vi "PH_PILS.set PPMA.vi"(0 "i ref in":refnum<vi>, 2 "Tagname":string="N/A", 5 "error in":errorcluster) -> (14 "i ref out":refnum<vi>, 19 "error out":errorcluster)   [LabVIEW 2014, in "PH_PILS.lvlib"]
doc: "Sets GUI elements related to PPMA."
uses:
  PH_PILS.lvlib
  PH_Common/PH_Common.lvlib
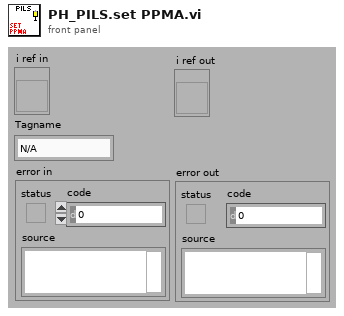
[diagram p1: front panel]
types:
  T1 = typedef "PH_PILS.lvlib/PH_PILS.i attribute.ctl" = cluster{"Boolean":cluster{"GUI Ref":refnum<vi>, "Status":i32}[], "GUI Refs Exp. Shutters":cluster{"1":refnum<vi>, "2":refnum<vi>, "3":refnum<vi>, "4":refnum<vi>}, "Tristate2Run GUI Refs":refnum<vi>[], "EO-Likes":cluster{"GUI Ref":refnum<vi>, "Status":i32}[], "Operation Mode":cluster{"Operation Mode":T2, "GUI":cluster{"Ref State":refnum<vi>, "Ref":refnum<vi>}, "Servicemode":cluster{"Tagname":string, "Status":i32}, "Labormode":cluster{"Tagname":string, "Status":i32}, "Searchmode":cluster{"Tagname":string, "Status":i32}, "Shotmode":cluster{"Tagname":string, "Status":i32}}, "Submode":cluster{"Submode":T3, "GUI":cluster{"Ref State":refnum<vi>, "Ref":refnum<vi>}, "Submode":cluster{"Tagname":string, "Status":i32}}, "Experiment":cluster{"Experiment":enum16{"unknown", "intern", "4 (Z6)", "3", "2", "1"}, "GUI":cluster{"Ref State":refnum<vi>, "Ref":refnum<vi>}, "intern":cluster{"Tagname":string, "Status":i32}, "Exp 4":cluster{"Tagname":string, "Status":i32}, "Exp 3":cluster{"Tagname":string, "Status":i32}, "Exp 2":cluster{"Tagname":string, "Status":i32}, "Exp 1":cluster{"Tagname":string, "Status":i32}}, "TristateNormal":cluster{"GUI Ref":refnum<vi>, "Status":i32}[], "Door Tags":cluster{"GUI Ref":refnum<vi>, "Status":i32}[], "GUIlessTags":cluster{"Name":string, "Status":i32}[], "Beamline GUI Refs":refnum<vi>[], "Special Boolean":cluster{"GUI Ref":refnum<vi>, "Status":i32}[], "Laserpower":cluster{"GUI Ref":refnum<vi>, "Status":i32}[], "Shutter":cluster{"GUI Ref":refnum<vi>, "Status":i32}[], "Tristate EO Like":cluster{"GUI Ref":refnum<vi>, "Status":i32}[], "PP":cluster{"GUI Ref":refnum<vi>, "Status":i32, "Head Ref":refnum<vi>, "Slider Ref":refnum<vi>}[], "Switch Knobs":cluster{"GUI Ref":refnum<vi>, "Status":i32}[], "Latch Knob GUI Refs":refnum<vi>[], "FailureCounter":i32, "Enabled Status":cluster{"Laser":i32, "PreAmp":i32, "MainAmp":i32}, "Mercury":refnum<vi>, "Instance Rods":string, "Logfile":path, "Beckhoff-Instance Internal":string, "Beckhoff-Instance External":string, "Enabling Rights":cluster{"Name":string, "Password":string, "PA?":bool, "MA?":bool, "Exp?":bool}[]}
  T2 = typedef "PH_PILS.lvlib/PH_PILS.Operation Mode.ctl" = enum16{"unknown", "Service", "Labor", "Search", "Shot"}
  T3 = typedef "PH_PILS.lvlib/PH_PILS.Submode.ctl" = enum16{"unknown", "HV-Normal", "HV-Test"}
  T4 = cluster{"GUI Ref":refnum<vi>, "Status":i32, "Head Ref":refnum<vi>, "Slider Ref":refnum<vi>}[]
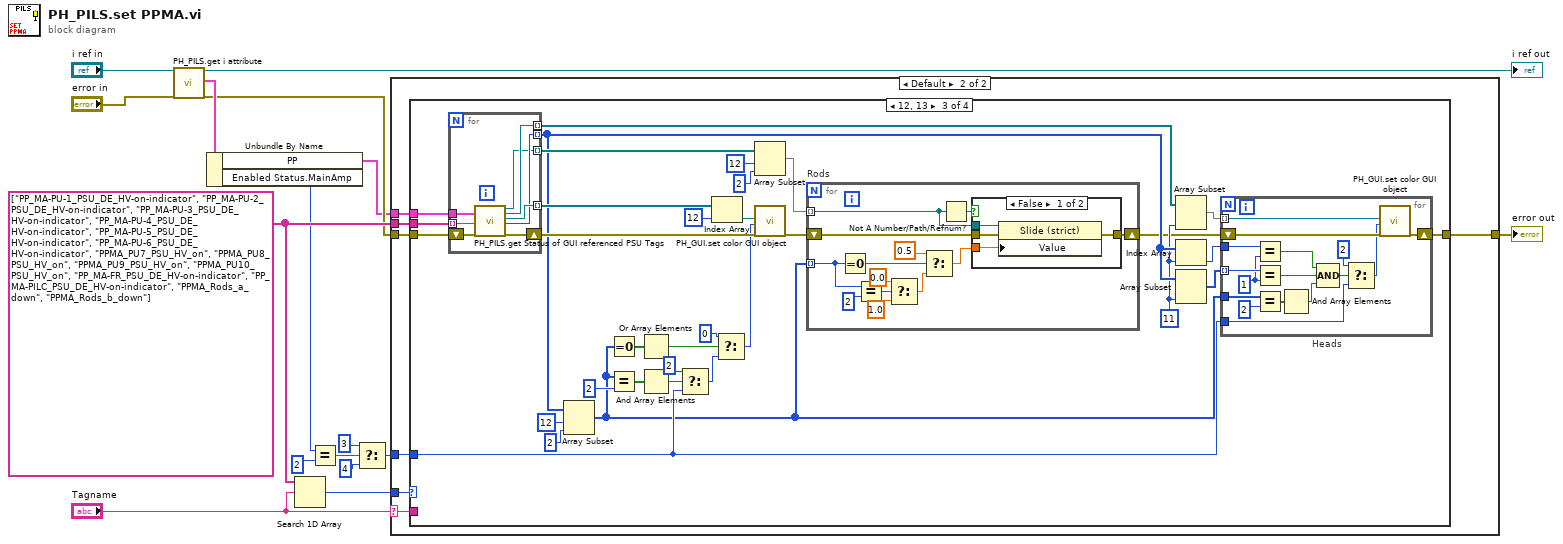
[diagram p0: block diagram]
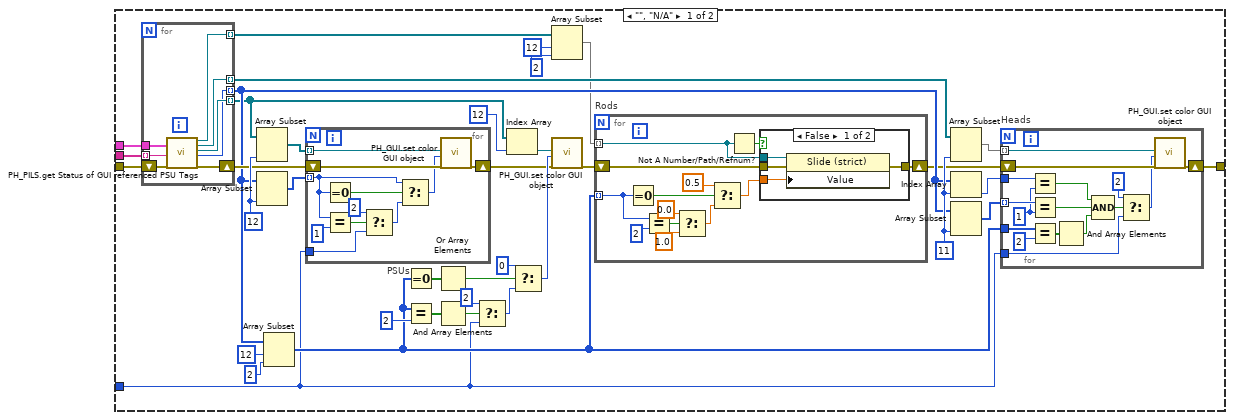
[diagram p2: hidden frame]
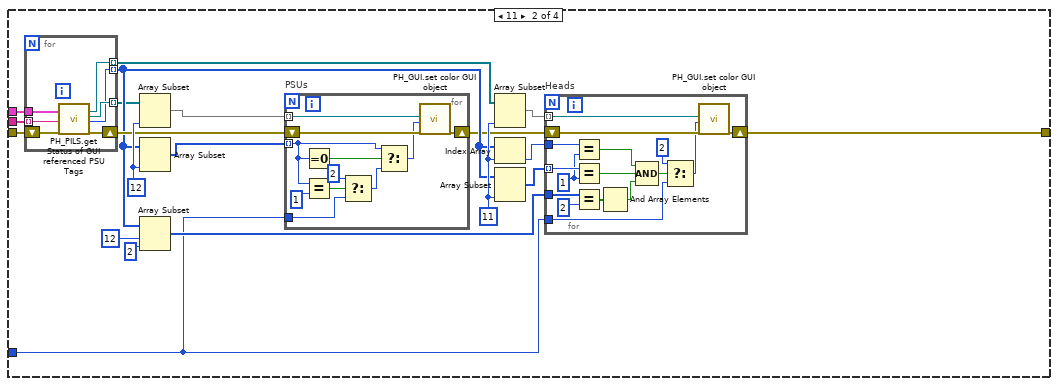
[diagram p5: hidden frame]
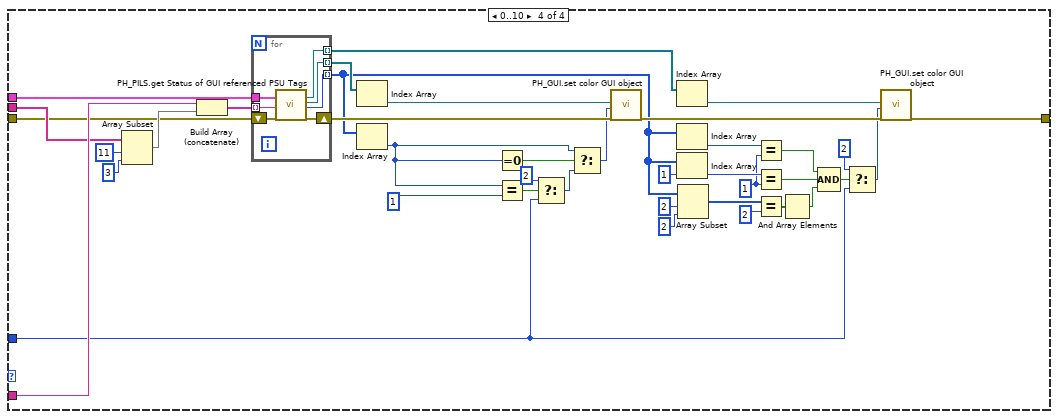
[diagram p7: hidden frame]
diagram:
  w15 = string[] ["PP_MA-PU-1_PSU_DE_HV-on-indicator", "PP_MA-PU-2_PSU_DE_HV-on-indicator", "PP_MA-PU-3_PSU_DE_HV-on-indicator", "PP_MA-PU-4_PSU_DE_HV-on-indicator", "PP_MA-PU-5_PSU_DE_HV-on-indicator", "PP_MA-PU-6_PSU_DE_HV-on-indicator", "PPMA_PU7_PSU_HV_on", "PPMA_PU8_PSU_HV_on", "PPMA_PU9_PSU_HV_on", "PPMA_PU10_PSU_HV_on", "PP_MA-FR_PSU_DE_HV-on-indicator", "PP_MA-PILC_PSU_DE_HV-on-indicator", "PPMA_Rods_a_down", "PPMA_Rods_b_down"]
  n1 = call "PH_PILS.get i attribute.vi"("i ref in"="i ref in", "error in (no error)"="error in") -> ("i ref out"=→"i ref out":refnum<vi>, "i attribute"=w12:T1, "error out"=w9:errorcluster)  [unwired: 15 in]
  n2 = Unbundle By Name(w12) -> ("PP"=w7:T4, "Enabled Status.MainAmp"=w2:i32)
  n3 = Search 1D Array(1D array=w15, element="Tagname") -> (index of element=w13:i32)  [unwired: 1 in]
  n4 = Equal?(x=w2, y=2 ("Status")) -> (x = y?=w3:bool)
  n5 = Select(t=3 ("Status"), s=w3, f=4 ("Status")) -> (s? t:f=w1:i32)
  n6 = case shown="Default" "Tagname" {
    selector: "Tagname" -> [_ w109]
    tunnel: w9 -> [w23 w111]
    tunnel: [w53 w107] -> w16
    tunnel: w15 -> [w24 w112]
    tunnel: w13 -> [_ w108]
    tunnel: w7 -> [w22 w113]
    tunnel: w1 -> [w21 w110]
    frame "", "N/A" {
      w33 = 11 ("length")
      w43 = 12 ("length")
      n7 = for {
        tunnel: w22 -> [w82]
        shift-right: [w87] -> w40
        shift-left: w23 -> [w88]
        tunnel: w24 -> [w83] mode=indexing
        tunnel: [w86] -> w39 mode=indexing
        tunnel: [w85] -> w29 mode=indexing
        tunnel: [w84] -> w30 mode=indexing
        tunnel: [w81] -> w18 mode=indexing
        n8 = call "PH_PILS.get Status of GUI referenced PSU Tags.vi"("PP Tag"=w82, "Tagname"=w83, "error in"=w88) -> ("Slider Ref"=w81:refnum<vi>, "Head Ref"=w86:refnum<vi>, "GUI Ref"=w85:refnum<vi>, "Status"=w84:i32, "error out"=w87:errorcluster)  [unwired: 11 in, 1 out]
      }
      n9 = Array Subset(array=w29, length=w43) -> (w41:refnum<vi>[])  [unwired: 1 in]
      n10 = Array Subset(array=w30, length=w43) -> (w42:i32[])  [unwired: 1 in]
      n11 = Array Subset(array=w30, index=12, length=2) -> (w26:i32[])
      n12 = for "PSUs" {
        shift-right: [w80] -> w28
        shift-left: w40 -> [w78]
        tunnel: w42 -> [w76] mode=indexing
        tunnel: w41 -> [w79] mode=indexing
        tunnel: w21 -> [w70]
        n13 = Equal To 0?(x=w76) -> (x = 0?=w77:bool)
        n14 = Equal?(x=w76, y=1) -> (x = y?=w74:bool)
        n15 = Select(t=2 ("y"), s=w74, f=w70) -> (s? t:f=w73:i32)
        n16 = Select(t=w76, s=w77, f=w73) -> (s? t:f=w71:i32)
        n17 = call "PH_GUI.set color GUI object.vi"("GUI object Ref"=w79, "State"=w71, "error in (no error)"=w78) -> ("error out"=w80:errorcluster)  [unwired: 16 in]
      }
      n18 = Equal To 0?(x=w26) -> (x = 0?=w52:bool[])
      n19 = Equal?(x=w26, y=2) -> (x = y?=w48:bool[])
      n20 = Or Array Elements(Boolean array=w52) -> (logical OR=w51:bool)
      n21 = And Array Elements(Boolean array=w48) -> (logical AND=w46:bool)
      n22 = Select(t=2 ("State"), s=w46, f=w21) -> (s? t:f=w45:i32)
      n23 = Index Array(array=w29, index=12) -> (element=w31:refnum<vi>)
      n24 = Select(t=0 ("State"), s=w51, f=w45) -> (s? t:f=w49:i32)
      n25 = Array Subset(array=w18, index=12, length=2) -> (w17:refnum<vi>[])
      n26 = call "PH_GUI.set color GUI object.vi"("GUI object Ref"=w31, "State"=w49, "error in (no error)"=w28) -> ("error out"=w27:errorcluster)  [unwired: 16 in]
      n27 = for "Rods" {
        shift-right: [w100] -> w25
        shift-left: w27 -> [w90]
        tunnel: w17 -> [w101] mode=indexing
        tunnel: w26 -> [w91] mode=indexing
        n28 = Equal To 0?(x=w91) -> (x = 0?=w99:bool)
        n29 = Equal?(x=w91, y=2) -> (x = y?=w95:bool)
        n30 = Select(t=0.0, s=w95, f=1.0) -> (s? t:f=w94:dbl)
        n31 = Select(t=0.5, s=w99, f=w94) -> (s? t:f=w98:dbl)
        n32 = Not A Number/Path/Refnum?(number/path/refnum=w101) -> (NaN/Path/Refnum?=w89:bool)
        n33 = case shown="False" w89 {
          tunnel: w90 -> [w102 w106]
          tunnel: [w105 w106] -> w100
          tunnel: w98 -> [w104 _]
          tunnel: w101 -> [w103 _]
          frame False {
            n34 = property class="Slide (strict)"(reference=w103, error in=w102, "Value"=w104) -> (error out=w105:errorcluster)  [unwired: 1 out]
          }
          frame True {
          }
        }
      }
      n35 = Array Subset(array=w39, length=w33) -> (w38:refnum<vi>[])  [unwired: 1 in]
      n36 = Index Array(array=w30, index=w33) -> (element=w36:i32)
      n37 = Array Subset(array=w30, length=w33) -> (w37:i32[])  [unwired: 1 in]
      n38 = for "Heads" {
        shift-right: [w69] -> w53
        shift-left: w25 -> [w66]
        tunnel: w38 -> [w68] mode=indexing
        tunnel: w37 -> [w67] mode=indexing
        tunnel: w36 -> [w65]
        tunnel: w26 -> [w64]
        tunnel: w21 -> [w57]
        w54 = 1 ("y")
        n39 = Equal?(x=w65, y=w54) -> (x = y?=w61:bool)
        n40 = Equal?(x=w67, y=w54) -> (x = y?=w55:bool)
        n41 = Equal?(x=w64, y=2 ("Status")) -> (x = y?=w62:bool[])
        n42 = And Array Elements(Boolean array=w62) -> (logical AND=w56:bool)
        n43 = Compound Arithmetic op=AND(w61, w55, w56) -> (w60:bool)
        n44 = Select(t=2 ("Status"), s=w60, f=w57) -> (s? t:f=w58:i32)
        n45 = call "PH_GUI.set color GUI object.vi"("GUI object Ref"=w68, "State"=w58, "error in (no error)"=w66) -> ("error out"=w69:errorcluster)  [unwired: 16 in]
      }
    }
    frame Default {
      n46 = case shown="12, 13" w108 {
        tunnel: w111 -> [w114 w117 w175 w246]
        tunnel: [w114 w119 w177 w282] -> w107
        tunnel: w112 -> [_ w120 w176 w267]
        tunnel: w109 -> [_ _ _ w270]
        tunnel: w113 -> [_ w116 w174 w245]
        tunnel: w110 -> [_ w115 w173 w244]
        frame Default {
        }
        frame 11 {
          w124 = 11 ("length")
          w134 = 12 ("length")
          n47 = for {
            tunnel: w116 -> [w162]
            shift-right: [w167] -> w131
            shift-left: w117 -> [w168]
            tunnel: w120 -> [w163] mode=indexing
            tunnel: [w166] -> w130 mode=indexing
            tunnel: [w165] -> w122 mode=indexing
            tunnel: [w164] -> w123 mode=indexing
            n48 = call "PH_PILS.get Status of GUI referenced PSU Tags.vi"("PP Tag"=w162, "Tagname"=w163, "error in"=w168) -> ("Head Ref"=w166:refnum<vi>, "GUI Ref"=w165:refnum<vi>, "Status"=w164:i32, "error out"=w167:errorcluster)  [unwired: 11 in, 2 out]
          }
          n49 = Array Subset(array=w122, length=w134) -> (w132:refnum<vi>[])  [unwired: 1 in]
          n50 = Array Subset(array=w123, length=w134) -> (w133:i32[])  [unwired: 1 in]
          n51 = Array Subset(array=w123, index=12, length=2) -> (w121:i32[])
          n52 = for "PSUs" {
            shift-right: [w161] -> w118
            shift-left: w131 -> [w159]
            tunnel: w133 -> [w157] mode=indexing
            tunnel: w132 -> [w160] mode=indexing
            tunnel: w115 -> [w151]
            n53 = Equal To 0?(x=w157) -> (x = 0?=w158:bool)
            n54 = Equal?(x=w157, y=1) -> (x = y?=w155:bool)
            n55 = Select(t=2 ("y"), s=w155, f=w151) -> (s? t:f=w154:i32)
            n56 = Select(t=w157, s=w158, f=w154) -> (s? t:f=w152:i32)
            n57 = call "PH_GUI.set color GUI object.vi"("GUI object Ref"=w160, "State"=w152, "error in (no error)"=w159) -> ("error out"=w161:errorcluster)  [unwired: 16 in]
          }
          n58 = Array Subset(array=w130, length=w124) -> (w129:refnum<vi>[])  [unwired: 1 in]
          n59 = Index Array(array=w123, index=w124) -> (element=w127:i32)
          n60 = Array Subset(array=w123, length=w124) -> (w128:i32[])  [unwired: 1 in]
          n61 = for "Heads" {
            shift-right: [w150] -> w119
            shift-left: w118 -> [w147]
            tunnel: w129 -> [w149] mode=indexing
            tunnel: w128 -> [w148] mode=indexing
            tunnel: w127 -> [w146]
            tunnel: w121 -> [w145]
            tunnel: w115 -> [w138]
            w135 = 1 ("y")
            n62 = Equal?(x=w146, y=w135) -> (x = y?=w142:bool)
            n63 = Equal?(x=w148, y=w135) -> (x = y?=w136:bool)
            n64 = Equal?(x=w145, y=2 ("Status")) -> (x = y?=w143:bool[])
            n65 = And Array Elements(Boolean array=w143) -> (logical AND=w137:bool)
            n66 = Compound Arithmetic op=AND(w142, w136, w137) -> (w141:bool)
            n67 = Select(t=2 ("Status"), s=w141, f=w138) -> (s? t:f=w139:i32)
            n68 = call "PH_GUI.set color GUI object.vi"("GUI object Ref"=w149, "State"=w139, "error in (no error)"=w147) -> ("error out"=w150:errorcluster)  [unwired: 16 in]
          }
        }
        frame 12, 13 {
          w193 = 11 ("length")
          n69 = for {
            tunnel: w174 -> [w237]
            shift-right: [w242] -> w201
            shift-left: w175 -> [w243]
            tunnel: w176 -> [w238] mode=indexing
            tunnel: [w241] -> w187 mode=indexing
            tunnel: [w240] -> w199 mode=indexing
            tunnel: [w239] -> w198 mode=indexing
            tunnel: [w236] -> w200 mode=indexing
            n70 = call "PH_PILS.get Status of GUI referenced PSU Tags.vi"("PP Tag"=w237, "Tagname"=w238, "error in"=w243) -> ("Slider Ref"=w236:refnum<vi>, "Head Ref"=w241:refnum<vi>, "GUI Ref"=w240:refnum<vi>, "Status"=w239:i32, "error out"=w242:errorcluster)  [unwired: 11 in, 1 out]
          }
          n71 = Array Subset(array=w198, index=12, length=2) -> (w170:i32[])
          n72 = Equal To 0?(x=w170) -> (x = 0?=w178:bool[])
          n73 = Equal?(x=w170, y=2) -> (x = y?=w182:bool[])
          n74 = Or Array Elements(Boolean array=w178) -> (logical OR=w179:bool)
          n75 = And Array Elements(Boolean array=w182) -> (logical AND=w184:bool)
          n76 = Select(t=2 ("State"), s=w184, f=w173) -> (s? t:f=w185:i32)
          n77 = Index Array(array=w199, index=12) -> (element=w195:refnum<vi>)
          n78 = Select(t=0 ("State"), s=w179, f=w185) -> (s? t:f=w181:i32)
          n79 = Array Subset(array=w200, index=12, length=2) -> (w172:refnum<vi>[])
          n80 = call "PH_GUI.set color GUI object.vi"("GUI object Ref"=w195, "State"=w181, "error in (no error)"=w201) -> ("error out"=w171:errorcluster)  [unwired: 16 in]
          n81 = for "Rods" {
            shift-right: [w213] -> w169
            shift-left: w171 -> [w203]
            tunnel: w172 -> [w214] mode=indexing
            tunnel: w170 -> [w204] mode=indexing
            n82 = Equal To 0?(x=w204) -> (x = 0?=w212:bool)
            n83 = Equal?(x=w204, y=2) -> (x = y?=w208:bool)
            n84 = Select(t=0.0, s=w208, f=1.0) -> (s? t:f=w207:dbl)
            n85 = Select(t=0.5, s=w212, f=w207) -> (s? t:f=w211:dbl)
            n86 = Not A Number/Path/Refnum?(number/path/refnum=w214) -> (NaN/Path/Refnum?=w202:bool)
            n87 = case shown="False" w202 {
              tunnel: w203 -> [w215 w219]
              tunnel: [w218 w219] -> w213
              tunnel: w211 -> [w217 _]
              tunnel: w214 -> [w216 _]
              frame False {
                n88 = property class="Slide (strict)"(reference=w216, error in=w215, "Value"=w217) -> (error out=w218:errorcluster)  [unwired: 1 out]
              }
              frame True {
              }
            }
          }
          n89 = Array Subset(array=w187, length=w193) -> (w188:refnum<vi>[])  [unwired: 1 in]
          n90 = Index Array(array=w198, index=w193) -> (element=w190:i32)
          n91 = Array Subset(array=w198, length=w193) -> (w189:i32[])  [unwired: 1 in]
          n92 = for "Heads" {
            shift-right: [w235] -> w177
            shift-left: w169 -> [w232]
            tunnel: w188 -> [w234] mode=indexing
            tunnel: w189 -> [w233] mode=indexing
            tunnel: w190 -> [w231]
            tunnel: w170 -> [w230]
            tunnel: w173 -> [w223]
            w220 = 1 ("y")
            n93 = Equal?(x=w231, y=w220) -> (x = y?=w227:bool)
            n94 = Equal?(x=w233, y=w220) -> (x = y?=w221:bool)
            n95 = Equal?(x=w230, y=2 ("Status")) -> (x = y?=w228:bool[])
            n96 = And Array Elements(Boolean array=w228) -> (logical AND=w222:bool)
            n97 = Compound Arithmetic op=AND(w227, w221, w222) -> (w226:bool)
            n98 = Select(t=2 ("Status"), s=w226, f=w223) -> (s? t:f=w224:i32)
            n99 = call "PH_GUI.set color GUI object.vi"("GUI object Ref"=w234, "State"=w224, "error in (no error)"=w232) -> ("error out"=w235:errorcluster)  [unwired: 16 in]
          }
        }
        frame 0..10 {
          w248 = 1 ("y")
          n100 = Array Subset(array=w267, index=11, length=3) -> (w266:string[])
          n101 = Build Array (concatenate)(w270, w266) -> (w265:string[])
          n102 = for {
            tunnel: w245 -> [w283]
            tunnel: [w288] -> w278 mode=indexing
            tunnel: [w287] -> w247 mode=indexing
            tunnel: [w286] -> w273 mode=indexing
            tunnel: w265 -> [w284] mode=indexing
            shift-right: [w289] -> w279
            shift-left: w246 -> [w285]
            n103 = call "PH_PILS.get Status of GUI referenced PSU Tags.vi"("PP Tag"=w283, "Tagname"=w284, "error in"=w285) -> ("Head Ref"=w288:refnum<vi>, "GUI Ref"=w286:refnum<vi>, "Status"=w287:i32, "error out"=w289:errorcluster)  [unwired: 11 in, 2 out]
          }
          n104 = Index Array(array=w273) -> (element=w280:refnum<vi>)  [unwired: 1 in]
          n105 = Index Array(array=w247) -> (element=w281:i32)  [unwired: 1 in]
          n106 = Equal To 0?(x=w281) -> (x = 0?=w264:bool)
          n107 = Equal?(x=w281, y=1) -> (x = y?=w262:bool)
          n108 = Select(t=2 ("y"), s=w262, f=w244) -> (s? t:f=w261:i32)
          n109 = Select(t=w281, s=w264, f=w261) -> (s? t:f=w259:i32)
          n110 = call "PH_GUI.set color GUI object.vi"("GUI object Ref"=w280, "State"=w259, "error in (no error)"=w279) -> ("error out"=w271:errorcluster)  [unwired: 16 in]
          n111 = Index Array(array=w278) -> (element=w277:refnum<vi>)  [unwired: 1 in]
          n112 = Index Array(array=w247) -> (element=w276:i32)  [unwired: 1 in]
          n113 = Index Array(array=w247, index=1) -> (element=w257:i32)
          n114 = Array Subset(array=w247, index=2, length=2) -> (w272:i32[])
          n115 = Equal?(x=w276, y=w248) -> (x = y?=w254:bool)
          n116 = Equal?(x=w257, y=w248) -> (x = y?=w249:bool)
          n117 = Equal?(x=w272, y=2 ("Status")) -> (x = y?=w255:bool[])
          n118 = And Array Elements(Boolean array=w255) -> (logical AND=w250:bool)
          n119 = Compound Arithmetic op=AND(w254, w249, w250) -> (w253:bool)
          n120 = Select(t=2 ("Status"), s=w253, f=w244) -> (s? t:f=w251:i32)
          n121 = call "PH_GUI.set color GUI object.vi"("GUI object Ref"=w277, "State"=w251, "error in (no error)"=w271) -> ("error out"=w282:errorcluster)  [unwired: 16 in]
        }
      }
    }
  }
  "error out" <- w16
